vi "LoadPreStartAttributes.vi"(8 "error in (no error)":errorcluster, 11 "SMO in":refnum<class "SMO.lvclass">) -> (0 "error out":errorcluster, 3 "SMO out":refnum<class "SMO.lvclass">)   [LabVIEW 2013, in "SMO.lvclass"]
uses:
  SMO.lvclass
  SMO.lvclass/SMO.ctl
  ReftoDVR--SMO.vi
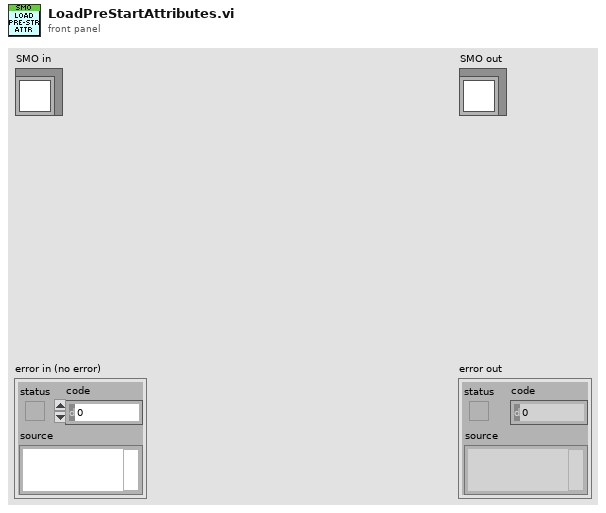
[diagram p1: front panel]
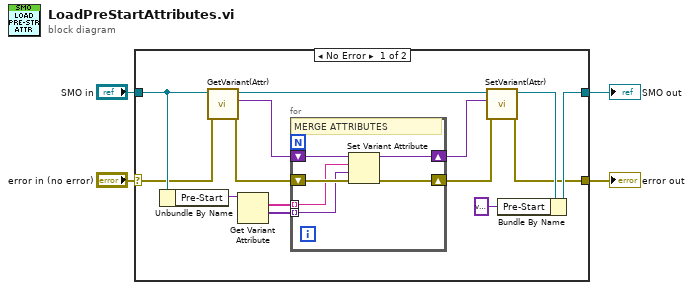
[diagram p0: block diagram]
diagram:
  n1 = case shown="No Error" "error in (no error)" {
    selector: "error in (no error)" -> [w11 w26]
    tunnel: [w10 w26] -> w3
    tunnel: [w18 w25] -> w1
    tunnel: "SMO in" -> [w15 w25]
    frame No Error {
      n2 = Unbundle By Name(w15) -> ("Pre-Start"=w14:variant)
      n3 = call "GetVariant(Attr).vi"("error in (no error)"=w11, "SMO in"=w15) -> ("error out"=w8:errorcluster, "[Attributes]"=w5:variant, "SMO out"=w9:refnum<class "SMO.lvclass">)  [unwired: 7 in]
      n4 = Get Variant Attribute(Variant=w14) -> (names=w13:string[], values=w12:variant[])  [unwired: 3 in, 2 out]
      n5 = for {
        tunnel: w13 -> [w20] mode=indexing
        tunnel: w12 -> [w19] mode=indexing
        shift-right: [w23] -> w7
        shift-left: w8 -> [w24]
        shift-right: [w22] -> w6
        shift-left: w5 -> [w21]
        # "MERGE ATTRIBUTES"
        n6 = Set Variant Attribute(Variant=w21, name=w20, value=w19, error in=w24) -> (Variant out=w22:variant, error out=w23:errorcluster)  [unwired: 1 out]
      }
      n7 = call "SetVariant(Attr).vi"("error in (no error)"=w7, "[Attributes]"=w6, "SMO in"=w9) -> ("error out"=w10:errorcluster, "SMO out"=w16:refnum<class "SMO.lvclass">)  [unwired: 7 in]
      n8 = Bundle By Name(cluster=w16, "Pre-Start"=variant) -> (w18:refnum<class "SMO.lvclass">)
    }
    frame Error {
    }
  }
  "error out" <- w3
  "SMO out" <- w1
